vi "serialization tests.vi"() -> (2 "modules equal":bool, 3 "channels equal":bool)   [LabVIEW 2014, in "UI reference module tests.lvlib"]
uses:
  UI reference module tests.lvlib
  module/configuration/UI Reference configuration old.lvclass
panel:
  out "data":string
  out "no error 2":errorcluster
  out "no error 1":errorcluster
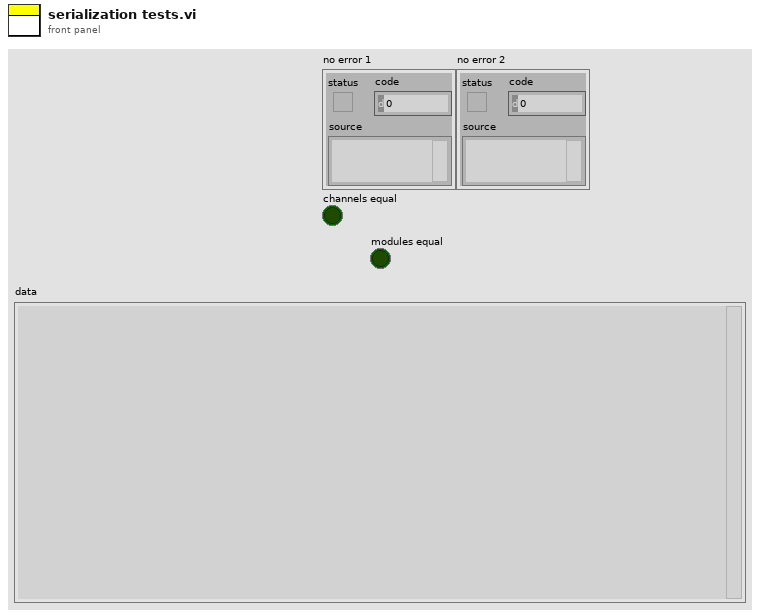
[diagram p1: front panel]
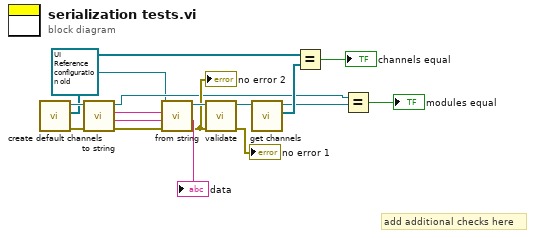
[diagram p0: block diagram]
diagram:
  # "add additional checks here"
  n1 = call "create default channels.vi"() -> ("error out"=w6:errorcluster, "channels"=w5:refnum<class "TBM channel.lvclass">[], "module"=w7:refnum<class "UI Reference configuration old.lvclass">)  [unwired: 7 in, 2 out]
  n2 = call-dynamic "to string.vi"("error in"=w6, "UI Reference configuration in"=w7) -> ("error out"=w16:errorcluster, "data"=w15:string, "version"=w14:string, "UI Reference configuration out"=w2:refnum<class "UI Reference configuration old.lvclass">)  [unwired: 6 in]
  "data" <- w15
  n3 = call-dynamic "from string.vi"("error in"=w16, "data"=w15, "version"=w14, "UI Reference configuration in"=refnum<class "UI Reference configuration old.lvclass"> refnum ("tag bus configurable plugin module configuration")) -> ("error out"=w11:errorcluster, "UI Reference configuration out"=w13:refnum<class "UI Reference configuration old.lvclass">)  [unwired: 6 in]
  "no error 2" <- w11
  n4 = call-dynamic "validate.vi"("error in"=w11, "UI Reference configuration in"=w13) -> ("error out"=→"no error 1":errorcluster, "UI Reference configuration out"=w9:refnum<class "UI Reference configuration old.lvclass">)  [unwired: 8 in]
  n5 = call-dynamic "get channels.vi"("UI Reference configuration in"=w9) -> ("channels"=w8:refnum<class "TBM channel.lvclass">[], "UI Reference configuration out"=w3:refnum<class "UI Reference configuration old.lvclass">)  [unwired: 9 in]
  n6 = Equal?(x=w5, y=w8) -> (x = y?=→"channels equal":bool)
  n7 = Equal?(x=w2, y=w3) -> (x = y?=→"modules equal":bool)
